vi "Set Formatter.vi"(10 "formatter":refnum<class "Formatter.lvclass">, 11 "handler in":refnum<class "Handler.lvclass">) -> (3 "handler out":refnum<class "Handler.lvclass">)   [LabVIEW 2024, in "Logging.lvlib" / "Handler.lvclass"]
uses:
  Handler.lvclass
  Handler.lvclass/Handler.ctl
  Formatters/Formatter/Formatter.lvclass
panel:
  # "Connector Pane"
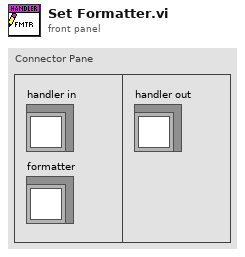
[diagram p1: front panel]
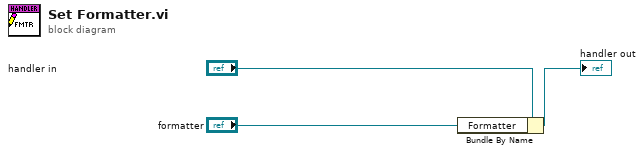
[diagram p0: block diagram]
diagram:
  n1 = Bundle By Name(cluster="handler in", "Formatter"="formatter") -> (→"handler out":refnum<class "Handler.lvclass">)
